vi "Remove_alpha_char.vi"(11 "input string":string) -> (3 "Result":string)   [LabVIEW 2019]
panel:
  out "length":i32
  out "substring":string
  in  "String chars":string="qwertyuiopasdfghjklzxcvbnmQWERTYUIOPASDFGHJKLZXCVBNM"
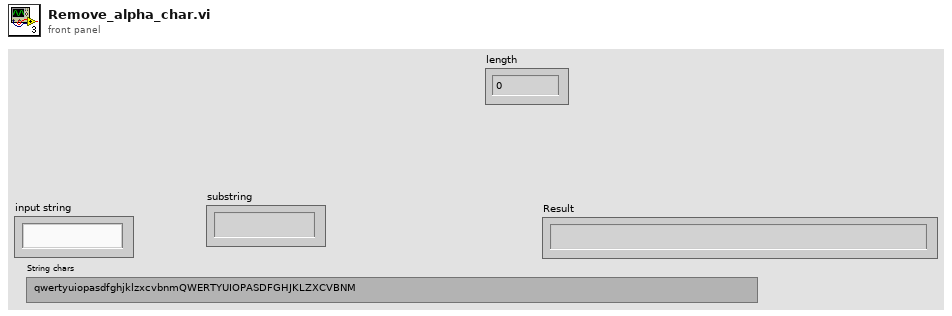
[diagram p1: front panel]
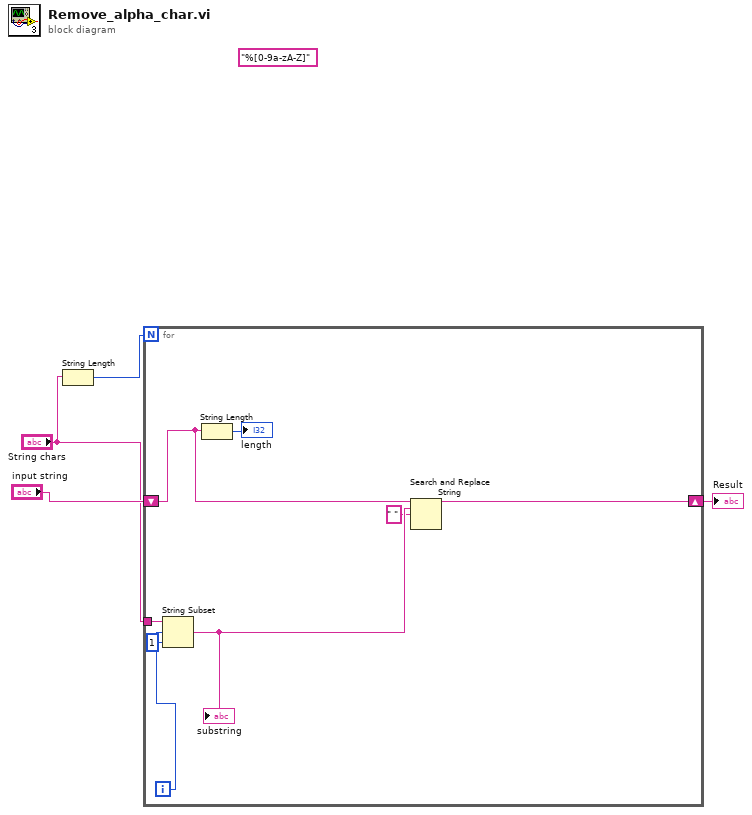
[diagram p0: block diagram]
diagram:
  (unwired) "%[0-9a-zA-Z]" ("format string")
  n1 = String Length(string="String chars") -> (length=w3:i32)
  n2 = for {
    N: w3 -> [_]
    tunnel: "String chars" -> [w12]
    shift-right: [w7] -> w1
    shift-left: "input string" -> [w8]
    i -> [w11]
    n3 = String Subset(string=w12, offset (0)=w11, length (rest)=1 ("length (rest)")) -> (substring=w6:string)
    "substring" <- w6
    n4 = String Length(string=w8) -> (length=→"length":i32)
    n5 = Search and Replace String(input string=w8, search string=w6, replace string=" " ("replace string (\"\")")) -> (result string=w7:string)  [unwired: 5 in, 3 out]
  }
  "Result" <- w1
